vi "XNET TCP Socket Read (Text).vi"(7 "mode (standard)":T1=1 items=["Standard"=1, "Buffered"=2, "CRLF"=3, "Immediate"=4], 8 "error in":errorcluster, 9 "timeout ms (25000)":i32=25000, 10 "bytes to read":i32, 11 "socket in":refnum<k20>) -> (0 "error out":errorcluster, 2 "data":string, 3 "socket out":refnum<k20>)   [LabVIEW 2018]
doc: "Reads a number of bytes from a TCP network connection and returns the results as string data."
uses:
  XNET TCP Socket Read Mode Text.ctl
  nixlvapi.dll
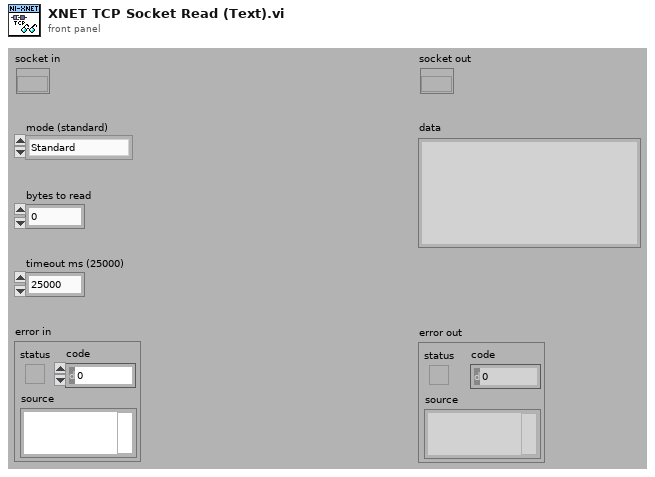
[diagram p1: front panel]
types:
  T1 = typedef "XNET TCP Socket Read Mode Text.ctl" = u32
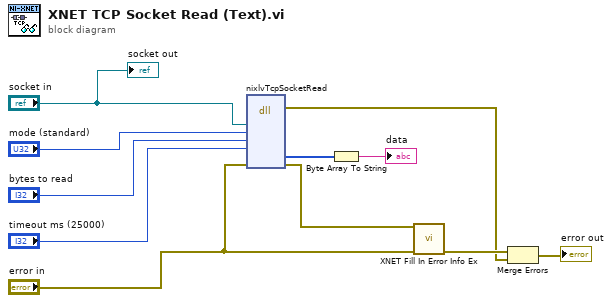
[diagram p0: block diagram]
diagram:
  n1 = dll-call lib="nixlvapi.*" fn="nixlvTcpSocketRead" label="Call Library"("socketRef"="socket in", "mode"="mode (standard)", "bytesToRead"="bytes to read", "timeoutMs"="timeout ms (25000)", "errorInOut"="error in") -> (error out=w8:errorcluster, "lvData"=w2:u8[], "errorInOut"=w10:errorcluster)  [unwired: 3 in, 7 out]
  n2 = Byte Array To String(unsigned byte array=w2) -> (string=→"data":string)
  n3 = call "XNET Fill In Error Info Ex.vi"("error xnet"=w10, "error in"="error in") -> ("error out"=w9:errorcluster)  [unwired: 13 in]
  n4 = Merge Errors(w9, w8) -> (→"error out":errorcluster)
  "socket out" <- "socket in"
